vi "Snap to Baseline.vi"(9 "Snap to baseline":bool, 10 "Point in":cluster{"x":dbl, "y":dbl, "th":dbl}, 11 "Picture in":refnum<vi>) -> (3 "Point out":cluster{"x":dbl, "y":dbl, "th":dbl})   [LabVIEW 2020]
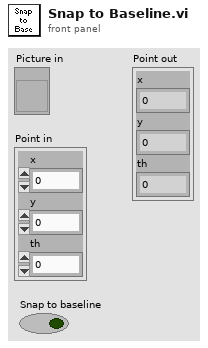
[diagram p1: front panel]
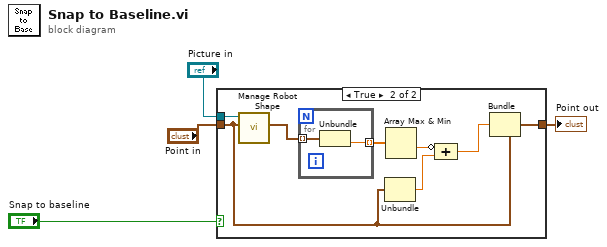
[diagram p0: block diagram]
diagram:
  n1 = case shown="True" "Snap to baseline" {
    tunnel: "Point in" -> [w5 w7]
    tunnel: [w5 w6] -> w3
    tunnel: "Picture in" -> [_ w11]
    frame False {
    }
    frame True {
      n2 = call "Manage Robot Shape.vi"("Robot Position (ft)"=w7, "Pict Ref"=w11) -> ("Boundary Poly"=w13:cluster{dbl, dbl}[])  [unwired: 7 in, 2 out]
      n3 = for {
        tunnel: w13 -> [w15] mode=indexing
        tunnel: [w14] -> w12 mode=indexing
        n4 = Unbundle(w15) -> (w14:dbl)  [unwired: 1 out]
      }
      n5 = Unbundle(w7) -> ("y"=w9:dbl)  [unwired: 2 out]
      n6 = Array Max & Min(array=w12) -> (min value=w10:dbl)  [unwired: 3 out]
      n7 = Compound Arithmetic op=ADD(invert w10, w9) -> (w8:dbl)
      n8 = Bundle(cluster=w7, "y"=w8) -> (w6:cluster{"x":dbl, "y":dbl, "th":dbl})  [unwired: 2 in]
    }
  }
  "Point out" <- w3
